vi "Test.vi"() -> ()   [LabVIEW 2019, in "BNT_SLTagConnection.lvlib"]
doc: "Test SystemLink implementation for derived class of CSPP_ProcessVariable.lvclass"
uses:
  BNT_SLTagConnection.lvlib
  CSPP_Core/Classes/CSPP_ProcessVariables/ProcessVariable/PV.lvclass
  BNT_SLTagConnection.lvclass
  C:/Users/Holger/Documents/LVP/CSPP/CSPP-Template/Packages/CSPP_Core/Classes/CSPP_ProcessVariables/PVConnection/PVConnection.lvclass
  CSPP_Core/Classes/CSPP_ProcessVariables/ProcessVariable/PV.lvclass/PV.ctl
  CSPP_Core/Classes/CSPP_ProcessVariables/PVConnection/PVConnection.lvclass/PVConnection.ctl
  CSPP_Core/Classes/CSPP_ProcessVariables/ProcessVariable/Read Timestamp.vi
  CSPP_Core/Classes/CSPP_ProcessVariables/ProcessVariable/Read Data.vi
  CSPP_Core/Classes/CSPP_ProcessVariables/ProcessVariable/Write Timestamp.vi
  CSPP_Core/Classes/CSPP_ProcessVariables/ProcessVariable/Write Data.vi
  CSPP_Core/Classes/CSPP_ProcessVariables/ProcessVariable/Write PV URL.vi
  CSPP_Core/Classes/CSPP_ProcessVariables/ProcessVariable/Write Type Descriptor.vi
  CSPP_Core/Classes/CSPP_ProcessVariables/ProcessVariable/Write Name.vi
  <vilib>/Utility/error.llb/Error Cluster From Error Code.vi
  <vilib>/regexp/Match Regular Expression.xnode
  CSPP_Core/Classes/CSPP_ProcessVariables/PVConnection/PVConnection.lvclass
panel:
  out "Receiver Iteration 1":i32
  in  "Receiver Interval 1":dbl[unit]=1.0
  out "Received 1":timestamp format="%<%x %.3X>T"
  out "Received Value 1":i32
  out "Received Value 0":i32
  out "Received 0":timestamp format="%<%x %.3X>T"
  out "Receiver Iteration 0":i32
  in  "Receiver Interval 0":dbl[unit]=1.0
  out "Published":timestamp format="%<%x %.3X>T"
  out "Published Value":i32
  in  "Publisher Interval":dbl[unit]=1.0
  in  "Stop":bool
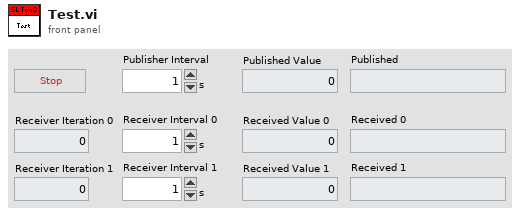
[diagram p1: front panel]
types:
  T1 = cluster{"Read Access":enum8{"Allowed", "Required", "None"}, "Write Access":enum8{"Allowed", "Required", "None"}}
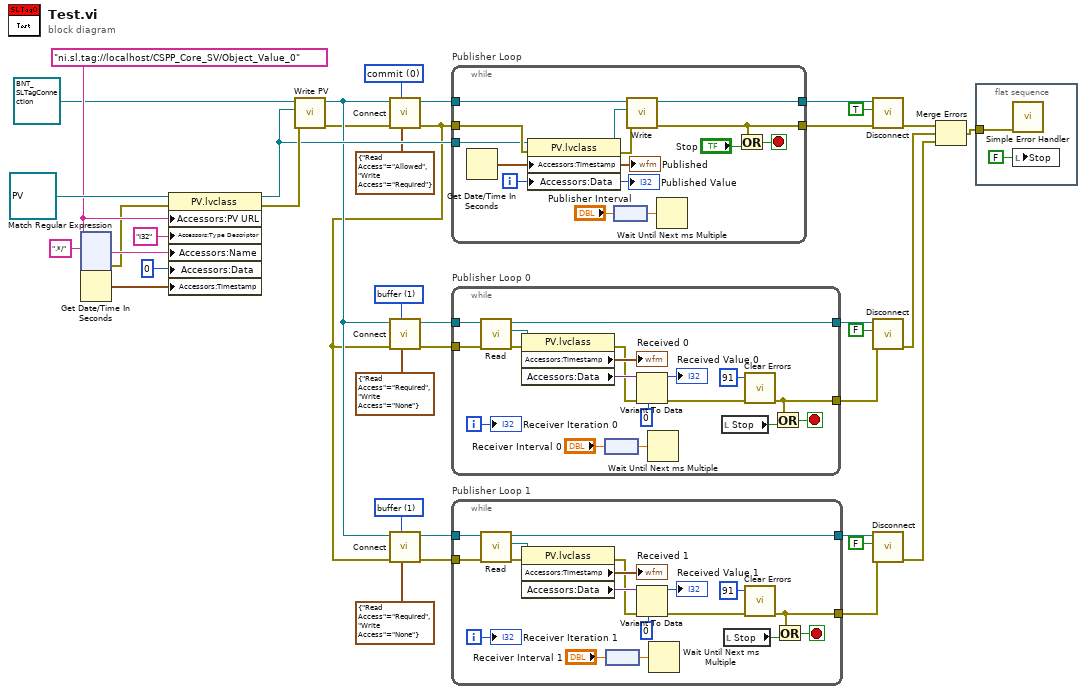
[diagram p0: block diagram]
diagram:
  w10 = u16 1 items=["commit", "buffer"] ("Mode (buffer)")
  w13 = u16 1 items=["commit", "buffer"] ("Mode (buffer)")
  w29 = u16 0 items=["commit", "buffer"] ("Mode (buffer)")
  w36 = "ni.sl.tag://localhost/CSPP_Core_SV/Object_Value_0" ("name (unnamed)")
  n1 = xnode "Match Regular Expression"("input string"=w36, "regular expression"=".*/") -> ("after match"=w35:string, "error out"=w31:errorcluster)  [unwired: 4 in, 3 out]
  n2 = Get Date/Time In Seconds() -> (seconds since 1Jan1904=w2:timestamp)
  n3 = property class="PV.lvclass"(reference=refnum<class "PV.lvclass"> refnum ("CSPP_ProcessVariables.lvlib:PV.lvclass"), error in=w31, "Accessors:PV URL"=w36, "Accessors:Type Descriptor"="I32" ("Type Descriptor"), "Accessors:Name"=w35, "Accessors:Data"=0, "Accessors:Timestamp"=w2) -> (reference out=w28:refnum<class "PV.lvclass">, error out=w32:errorcluster)
  n4 = call "Write PV.vi"("error in (no error)"=w32, "PV"=w28, "PVConnection in"=refnum<class "BNT_SLTagConnection.lvclass"> refnum ("BNT_SLTagConnection.lvlib:BNT_SLTagConnection.lvclass")) -> ("error out"=w20:errorcluster, "PVConnection out"=w21:refnum<class "BNT_SLTagConnection.lvclass">)  [unwired: 7 in]
  n5 = call "Connect.vi"("Access (R/W allowed)"=T1 {"Read Access"=enum."Allowed", "Write Access"=enum."Required"}, "Mode (buffer)"=w29, "Error In"=w20, "PVConnection in"=w21) -> ("Error Out"=w4:errorcluster, "PVConnection out"=w30:refnum<class "BNT_SLTagConnection.lvclass">)  [unwired: 6 in]
  n6 = call "Connect.vi"("Access (R/W allowed)"=T1 {"Read Access"=enum."Required", "Write Access"=enum."None"}, "Mode (buffer)"=w13, "Error In"=w4, "PVConnection in"=w21) -> ("Error Out"=w14:errorcluster, "PVConnection out"=w12:refnum<class "BNT_SLTagConnection.lvclass">)  [unwired: 6 in]
  n7 = call "Connect.vi"("Access (R/W allowed)"=T1 {"Read Access"=enum."Required", "Write Access"=enum."None"}, "Mode (buffer)"=w10, "Error In"=w4, "PVConnection in"=w21) -> ("Error Out"=w9:errorcluster, "PVConnection out"=w11:refnum<class "BNT_SLTagConnection.lvclass">)  [unwired: 6 in]
  n8 = while "Publisher Loop" {
    tunnel: w30 -> [w51]
    tunnel: w4 -> [w49]
    tunnel: w28 -> [w48]
    tunnel: [w41] -> w27
    tunnel: [w40] -> w26
    i -> [w44]
    stop <- w45 stop-if-true
    n9 = Get Date/Time In Seconds() -> (seconds since 1Jan1904=w39:timestamp)
    "Published" <- w39
    n10 = property class="PV.lvclass"(reference=w48, error in=w49, "Accessors:Timestamp"=w39, "Accessors:Data"=w44) -> (reference out=w47:refnum<class "PV.lvclass">, error out=w50:errorcluster)
    n11 = node("Publisher Interval") -> (w42:dbl)
    n12 = call "Write.vi"("error in (no error)"=w50, "PV"=w47, "PVConnection in"=w51) -> ("error out"=w40:errorcluster, "PVConnection out"=w41:refnum<class "BNT_SLTagConnection.lvclass">)  [unwired: 6 in, 1 out]
    n13 = Wait Until Next ms Multiple(millisecond multiple=w42) -> ()  [unwired: 1 out]
    n14 = Or(x=w40, y="Stop") -> (x .or. y?=w45:bool)
    "Published Value" <- w44
  }
  n15 = while "Publisher Loop 0" {
    tunnel: w12 -> [w66]
    tunnel: w14 -> [w64]
    tunnel: [w65] -> w15
    tunnel: [w53] -> w16
    i -> [w68]
    stop <- w69 stop-if-true
    n16 = call "Read.vi"("error in (no error)"=w64, "PVConnection in"=w66) -> ("error out"=w62:errorcluster, "PV"=w63:refnum<class "PV.lvclass">, "PVConnection out"=w65:refnum<class "BNT_SLTagConnection.lvclass">)  [unwired: 6 in, 1 out]
    n17 = property class="PV.lvclass"(reference=w63, error in=w62) -> (error out=w58:errorcluster, "Accessors:Timestamp"=→"Received 0":timestamp, "Accessors:Data"=w60:variant)  [unwired: 1 out]
    n18 = node("Receiver Interval 0") -> (w55:dbl)
    n19 = Variant To Data(error in=w58, type=0, Variant=w60) -> (data=→"Received Value 0":i32, error out=w57:errorcluster)
    n20 = Wait Until Next ms Multiple(millisecond multiple=w55) -> ()  [unwired: 1 out]
    n21 = local read "Stop"() -> (w67:bool)
    n22 = call <vilib>:"Clear Errors.vi"("error in (no error)"=w57, "specific error code to clear (0: all)"=91) -> ("error out"=w53:errorcluster)  [unwired: 4 in, 1 out]
    n23 = Or(x=w53, y=w67) -> (x .or. y?=w69:bool)
    "Receiver Iteration 0" <- w68
  }
  n24 = while "Publisher Loop 1" {
    tunnel: w11 -> [w84]
    tunnel: w9 -> [w82]
    tunnel: [w83] -> w8
    tunnel: [w71] -> w7
    i -> [w86]
    stop <- w87 stop-if-true
    n25 = call "Read.vi"("error in (no error)"=w82, "PVConnection in"=w84) -> ("error out"=w80:errorcluster, "PV"=w81:refnum<class "PV.lvclass">, "PVConnection out"=w83:refnum<class "BNT_SLTagConnection.lvclass">)  [unwired: 6 in, 1 out]
    n26 = property class="PV.lvclass"(reference=w81, error in=w80) -> (error out=w76:errorcluster, "Accessors:Timestamp"=→"Received 1":timestamp, "Accessors:Data"=w78:variant)  [unwired: 1 out]
    n27 = node("Receiver Interval 1") -> (w73:dbl)
    n28 = Variant To Data(error in=w76, type=0, Variant=w78) -> (data=→"Received Value 1":i32, error out=w75:errorcluster)
    n29 = Wait Until Next ms Multiple(millisecond multiple=w73) -> ()  [unwired: 1 out]
    n30 = local read "Stop"() -> (w85:bool)
    n31 = call <vilib>:"Clear Errors.vi"("error in (no error)"=w75, "specific error code to clear (0: all)"=91) -> ("error out"=w71:errorcluster)  [unwired: 4 in, 1 out]
    n32 = Or(x=w71, y=w85) -> (x .or. y?=w87:bool)
    "Receiver Iteration 1" <- w86
  }
  n33 = call "Disconnect.vi"("error in (no error)"=w26, "Force (T)"=TRUE, "PVConnection in"=w27) -> ("error out"=w24:errorcluster)  [unwired: 7 in, 1 out]
  n34 = call "Disconnect.vi"("error in (no error)"=w16, "Force (T)"=FALSE, "PVConnection in"=w15) -> ("error out"=w22:errorcluster)  [unwired: 7 in, 1 out]
  n35 = call "Disconnect.vi"("error in (no error)"=w7, "Force (T)"=FALSE, "PVConnection in"=w8) -> ("error out"=w19:errorcluster)  [unwired: 7 in, 1 out]
  n36 = Merge Errors(w24, w22, w19) -> (w38:errorcluster)
  n37 = flat-sequence {
    tunnel: w38 -> [w89]
    frame #0 {
      n38 = call <vilib>:"Simple Error Handler.vi"("error in (no error)"=w89) -> ()  [unwired: 4 in, 5 out]
      n39 = local write "Stop"(FALSE ("Stop")) -> ()
    }
  }
